vi "APSxSensorWriteData.vi"(8 "error in (no error)":errorcluster caption="错误输入（无错误）", 11 "hSENSOR":i32) -> (0 "error out":errorcluster caption="错误输出", 2 "Message":string, 3 "hSENSOR out":i32)   [LabVIEW 2020]
doc: "该模板用于创建子VI。"
uses:
  APSx.dll/APSx.dll
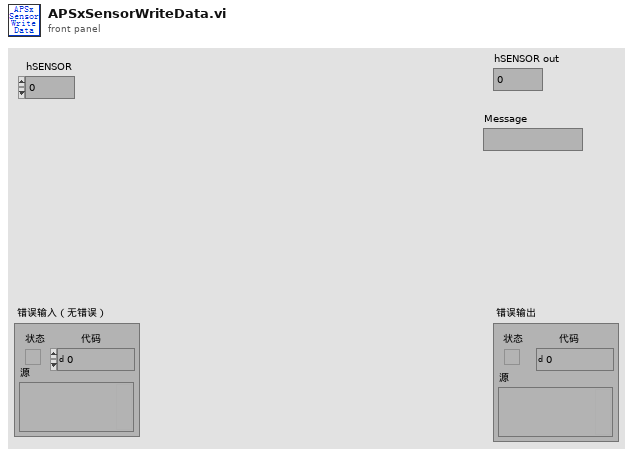
[diagram p1: front panel]
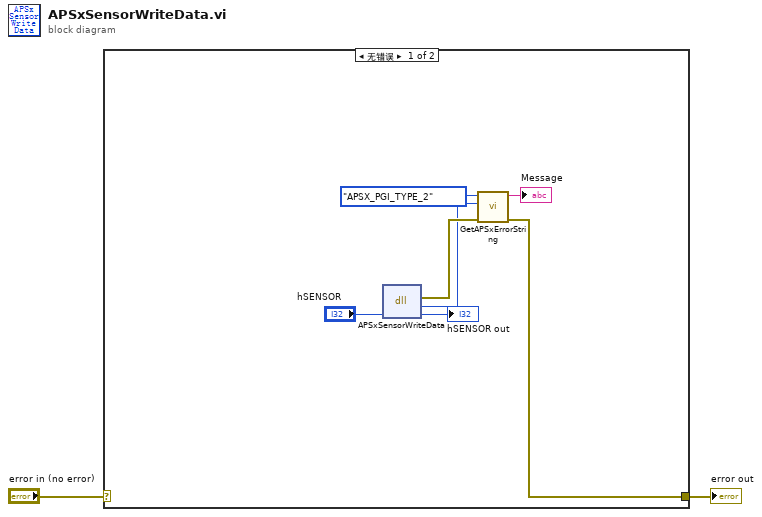
[diagram p0: block diagram]
diagram:
  n1 = case shown="无错误" "error in (no error)" {
    selector: "error in (no error)" -> [_ w10]
    tunnel: [w5 w10] -> w1
    frame No Error {
      n2 = dll-call lib="PTH2iabs CUsersFengDesktop传感器对中台传感器对中台labviewSourcesAPSx.dllAPSx.dll" fn="APSxSensorWriteData"("hSENSOR"="hSENSOR") -> (error out=w8:errorcluster, "Code"=w7:i32, "hSENSOR"=→"hSENSOR out":i32)  [unwired: 3 in, 1 out]
      n3 = call "GetAPSxErrorString.vi"("error in (no error)"=w8, "ErrorCode"=w7, "PGIType"=enum16{"APSX_PGI_TYPE_1", "APSX_PGI_TYPE_2"}."APSX_PGI_TYPE_2") -> ("error out"=w5:errorcluster, "Message"=→"Message":string)  [unwired: 7 in]
    }
    frame Error {
    }
  }
  "error out" <- w1
